vi "BuildLineNumbers.vi"(11 "Python Code":string) -> (3 "String":string)   [LabVIEW 2022 SP3]
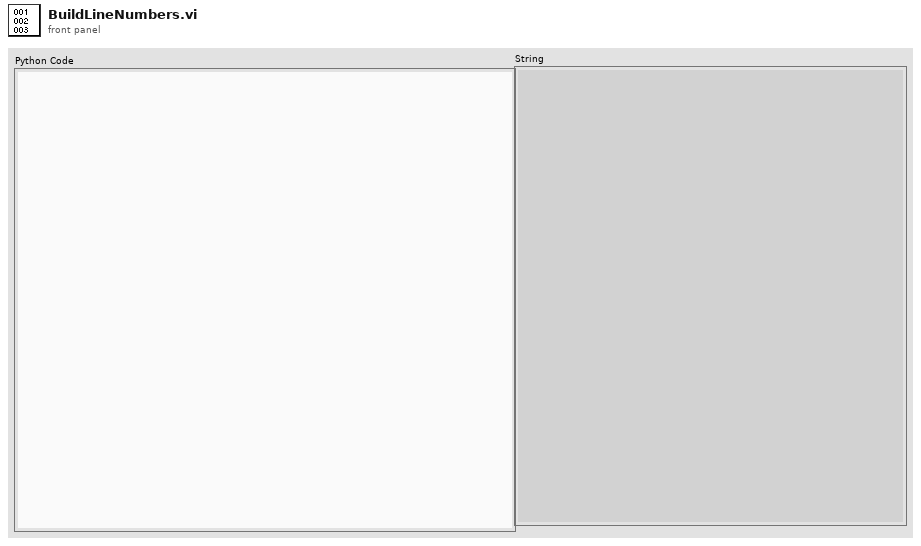
[diagram p1: front panel]
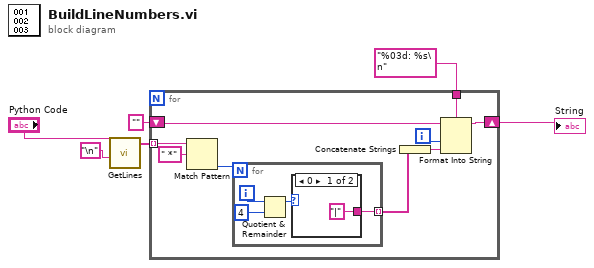
[diagram p0: block diagram]
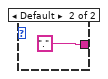
[diagram p2: hidden frame]
diagram:
  n1 = call "GetLines.vi"("delimiter"="\n", "String"="Python Code") -> ("Array"=w5:string[])  [unwired: 9 in]
  n2 = for {
    tunnel: "%03d: %s\n" ("format string") -> [w14]
    shift-right: [w13] -> w2
    shift-left: "" -> [w12]
    tunnel: w5 -> [w11] mode=indexing
    i -> [w15]
    n3 = Match Pattern(string=w11, regular expression=" *") -> (offset past match=w9:i32)  [unwired: 1 in, 3 out]
    n4 = for {
      N: w9 -> [_]
      tunnel: [w19] -> w8 mode=indexing
      i -> [w18]
      n5 = Quotient & Remainder(x=w18, y=4) -> (x-y*floor(x/y)=w17:i32)  [unwired: 1 out]
      n6 = case shown="0" w17 {
        tunnel: ["|" "."] -> w19
        frame 0 {
        }
        frame Default {
        }
      }
    }
    n7 = Concatenate Strings(w8) -> (w7:string)
    n8 = Format Into String(format string=w14, initial string=w12, w15, w7) -> (resulting string=w13:string)  [unwired: 1 in, 1 out]
  }
  "String" <- w2
